vi "To DVR.vi"(11 "Node":refnum<class "Node.lvclass">) -> (3 "DVR":refnum<data-value>)   [LabVIEW 2021, in "d20.lvlib" / "Node.lvclass"]
uses:
  Node.lvclass
  C:/Projects/lv2021-advent-of-code-2022/d20/INode/INode.lvclass
  INode/INode.lvclass
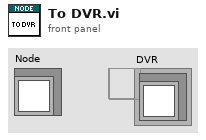
[diagram p1: front panel]
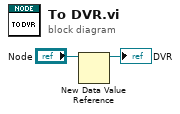
[diagram p0: block diagram]
diagram:
  n1 = New Data Value Reference(data value="Node") -> (data value reference=→"DVR":refnum<data-value>)  [unwired: 1 in, 1 out]
